vi "Write to Std In.vi"   [LabVIEW 2020, in "ase.lvlib" / "ase.lvclass"]
doc: "<B>Write data (raw bytes) or a String terminated with a newline to the standard input.</B>\n\nThis VI generates the following errors:\n-5691000: Internal Library Error. Check Error Message for more details.\n1556: Invalid Handle Supplied"
uses:
  ase.lvclass
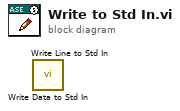
[diagram p0: block diagram]
diagram:
  n1 = call "Write Data to Std In.vi"() -> ()  [unwired: 9 in, 3 out]
  n2 = call "Write Line to Std In .vi"() -> ()  [unwired: 9 in, 3 out]
